vi "Lvi Subsystem Set Ctr Period Mode.vi"(8 "error in (no error)":errorcluster, 10 "InputLine":i32, 11 "TaskRef":i32) -> (0 "error out":errorcluster, 2 "function return":i32, 3 "TaskRef out":i32)   [LabVIEW 2016, in "DtLvLink.lvlib"]
doc: "Calls directly into the entry points of the DLL of the Data Acq SDK to create one or more virtual channels, add them to a task, and configure the task with the specified settings to measure the period, in milliseconds, of an external digital signal that is connected to the counter/timer's clock input or gate input source. This VI is used by the higher-level VI, DtOLCreateTask."
uses:
  <userlib>/LV-Link3/DtLvLink.lvlib
  <userlib>/LV-Link3/DtLvLink_32.dll
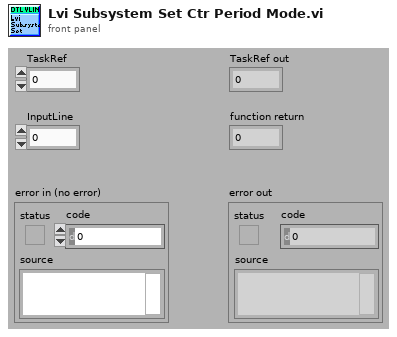
[diagram p1: front panel]
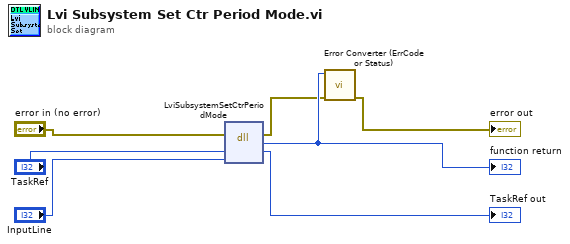
[diagram p0: block diagram]
diagram:
  n1 = dll-call lib="C:/Program Files (x86)/National Instruments/LabVIEW 2016/user.lib/LV-Link3/DtLvLink_32.*" fn="LviSubsystemSetCtrPeriodMode"(error in="error in (no error)", "TaskRef"="TaskRef", "InputLine"="InputLine") -> (error out=w2:errorcluster, w7:i32, "TaskRef"=→"TaskRef out":i32)  [unwired: 3 in, 1 out]
  "function return" <- w7
  n2 = call <userlib>:"Error Converter (ErrCode or Status).vi"("error in (no error)"=w2, "error code"=w7) -> ("error out"=→"error out":errorcluster)  [unwired: 9 in]
